vi "Exclude Path Options.vi"(8 "Error In":errorcluster, 11 "Path In":path) -> (0 "Error Out":errorcluster)   [LabVIEW 2010]
doc: "Use this template to build a standard state machine design pattern. Each state executes code and determines which state to transition to. Contrast this design pattern with the User Interface Event Handler pattern, in which code executes in response to user actions. Contrast this design pattern also with the Queued Message Handler pattern, in which each message handling code can queue zero or more new messages."
uses:
  Settings_option.ctl
panel:
  in  "System Key":string
  in  "EXCLUDE PATHS":path[](array[path])
  in  "Save":bool
  in  "Exit":bool
  # "OPTIONS"
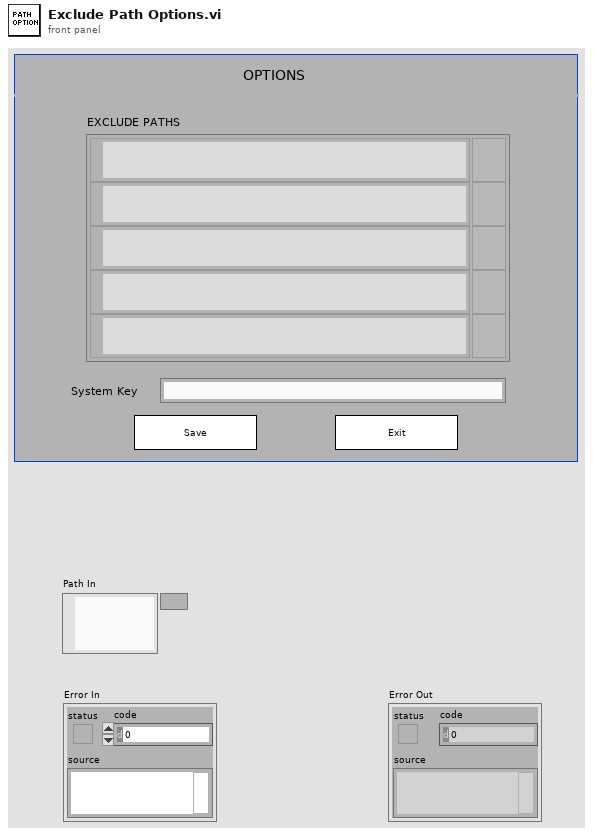
[diagram p1: front panel]
types:
  T1 = cluster{"Path In":path, "Exclude path":path[], "SystemKey":string}
  T2 = typedef "Settings_option.ctl" = enum16{"Poll", "Initialize", "Read", "Write", "Delete", "Exit"}
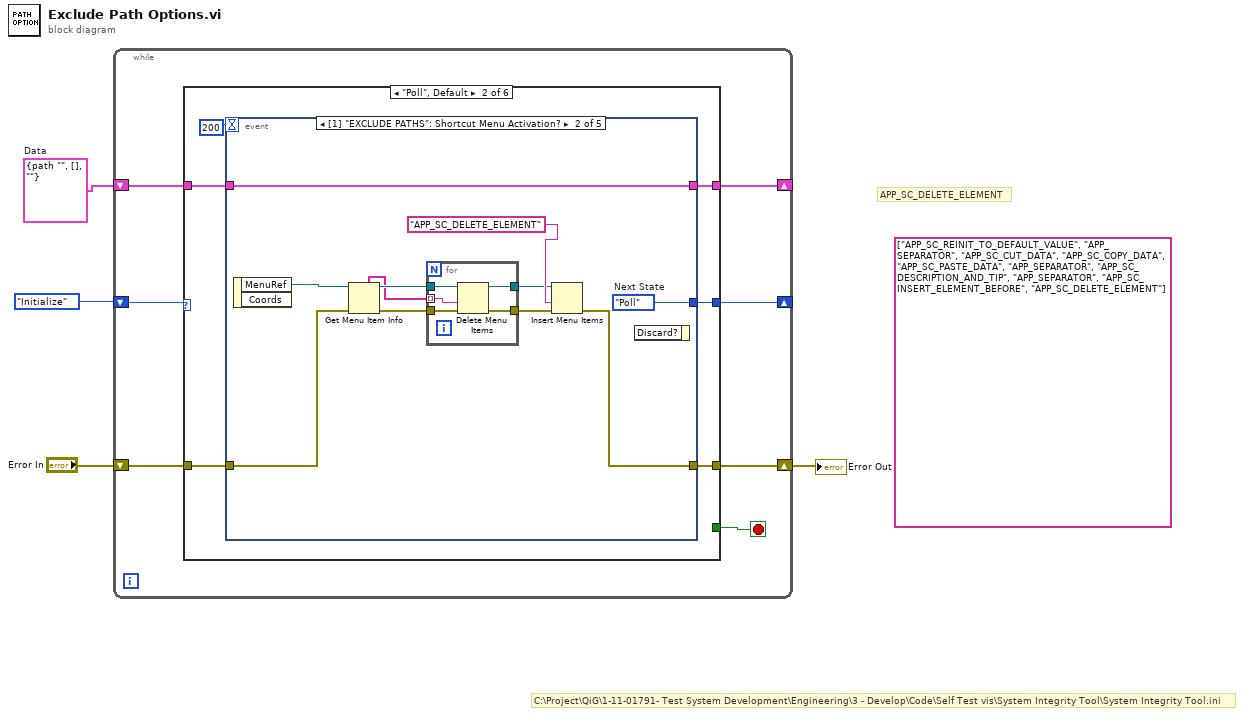
[diagram p0: block diagram]
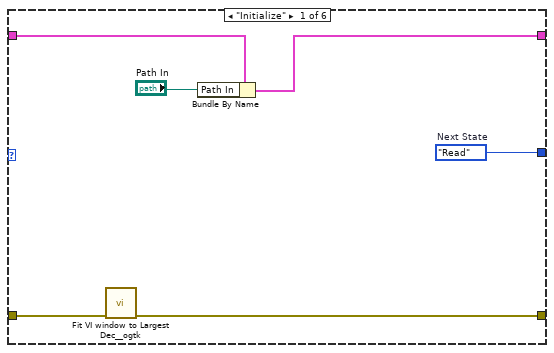
[diagram p2: hidden frame]
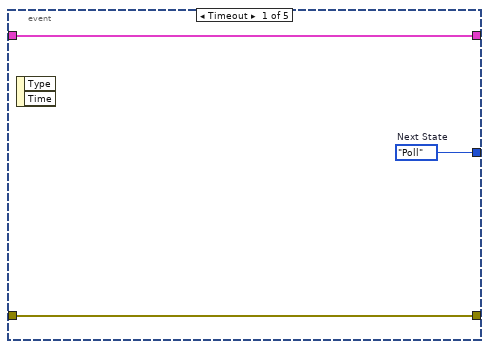
[diagram p3: hidden frame]
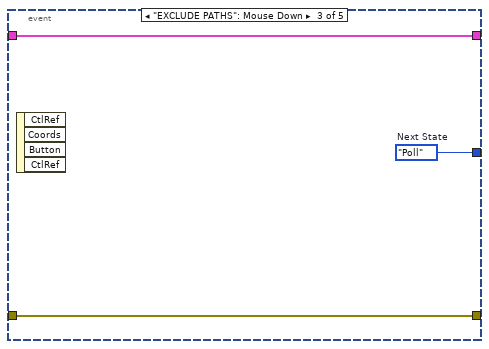
[diagram p4: hidden frame]
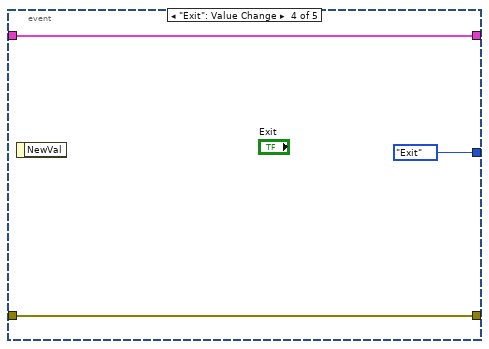
[diagram p5: hidden frame]
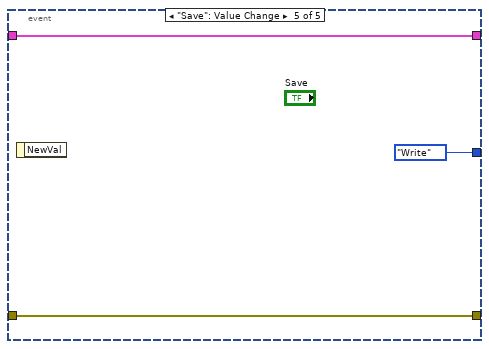
[diagram p6: hidden frame]
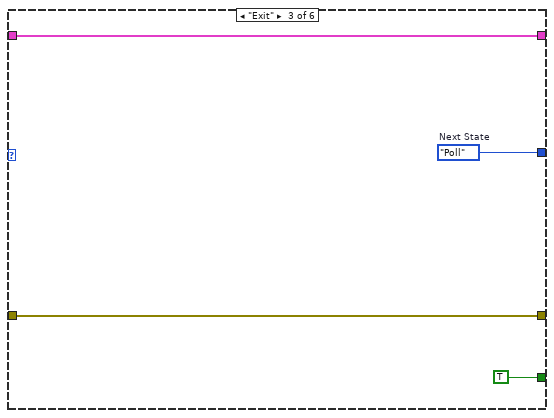
[diagram p7: hidden frame]
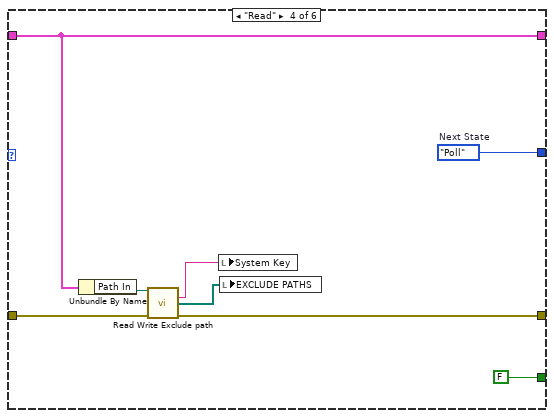
[diagram p8: hidden frame]
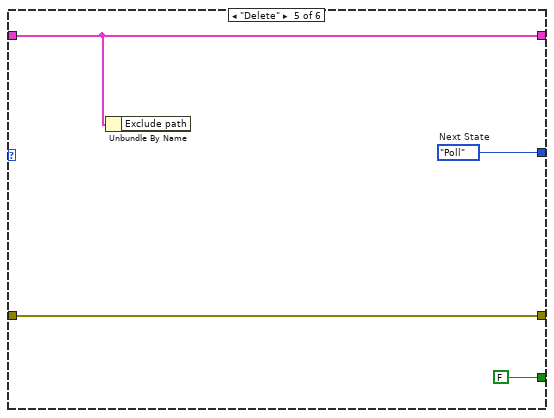
[diagram p9: hidden frame]
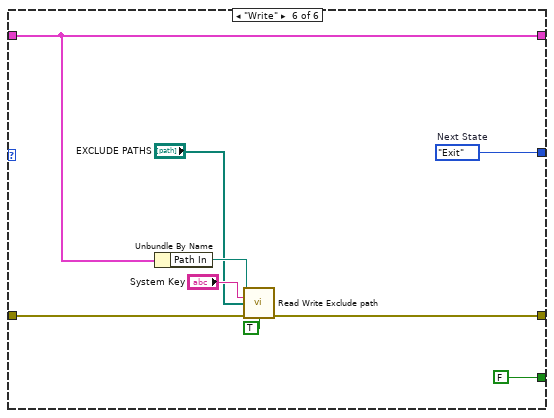
[diagram p10: hidden frame]
diagram:
  (unwired) string[] ["APP_SC_REINIT_TO_DEFAULT_VALUE", "APP_SEPARATOR", "APP_SC_CUT_DATA", "APP_SC_COPY_DATA", "APP_SC_PASTE_DATA", "APP_SEPARATOR", "APP_SC_DESCRIPTION_AND_TIP", "APP_SEPARATOR", "APP_SC_INSERT_ELEMENT_BEFORE", "APP_SC_DELETE_ELEMENT"] ("submenu tags 2")
  w1 = T1 {"Path In"=path "", "Exclude path"=[], "SystemKey"=""}  # Data
  # "APP_SC_DELETE_ELEMENT"
  # "C:\\Project\\QiG\\1-11-01791- Test System Development\\Engineering\\3 - Develop\\Code\\Self Test vis\\System Integrity Tool\\System Integrity Tool.ini"
  n1 = while {
    shift-right: [w10] -> _
    shift-left: Settings_option."Initialize" ("Beginning State") -> [w11]
    shift-right: [w7] -> w2
    shift-left: "Error In" -> [w8]
    shift-right: [w6] -> _
    shift-left: w1 -> [w5]
    stop <- w9 stop-if-true
    n2 = case shown="\"Poll\", Default" w11 {
      tunnel: [w17 w23 w55 w63 w67 w76] -> w10
      tunnel: [_ _ TRUE FALSE FALSE FALSE] -> w9
      tunnel: w8 -> [w16 w21 w53 w61 w64 w74]
      tunnel: [w15 w20 w53 w60 w64 w73] -> w7
      tunnel: [w13 w18 w52 w59 w65 w72] -> w6
      tunnel: w5 -> [w14 w19 w52 w59 w65 w72]
      frame "Initialize" {
        w17 = Settings_option."Read"  # Next State
        n3 = call "Fit VI window to Largest Dec__ogtk.vi"("error in (no error)"=w16) -> ("error out"=w15:errorcluster)  [unwired: 5 in, 1 out]
        n4 = Bundle By Name(cluster=w14, "Path In"="Path In") -> (w13:T1)
      }
      frame "Poll", Default {
        n5 = event shown="[1] \"EXCLUDE PATHS\": Shortcut Menu Activation?" {
          selector: _ -> [_ _ _ _ _]
          dyn-events: _ -> [_ _ _ _ _]
          timeout: 200 -> [_ _ _ _ _]
          tunnel: [w26 w37 w45 Settings_option."Exit" ("Next State") Settings_option."Write" ("Next State")] -> w23
          tunnel: [w25 w29 w44 w47 w50] -> w20
          tunnel: w21 -> [w25 w32 w44 w47 w50]
          tunnel: [w24 w36 w43 w46 w49] -> w18
          tunnel: w19 -> [w24 w36 w43 w46 w49]
          event Timeout {
            w26 = Settings_option."Poll"  # Next State
            n6 = event-data() -> ()  [unwired: 1 in, 2 out]
          }
          event "EXCLUDE PATHS": Shortcut Menu Activation? {
            w37 = Settings_option."Poll"  # Next State
            n7 = event-data() -> ("MenuRef"=w35:refnum<k9>)  [unwired: 1 in, 1 out]
            n8 = Get Menu Item Info(8:w32, 11:w35) -> (0:w33:errorcluster, 3:w34:refnum<k9>, 5:w31:string[])  [unwired: 1 in, 4 out]
            n9 = for {
              tunnel: w34 -> [w42]
              tunnel: w33 -> [w41]
              tunnel: w31 -> [w40] mode=indexing
              tunnel: [w39] -> w30
              tunnel: [w38] -> w27
              n10 = Delete Menu Items(6:w41, 7:w40, 9:w42) -> (0:w39:errorcluster, 3:w38:refnum<k9>)  [unwired: 1 in]
            }
            n11 = Insert Menu Items(6:w30, 7:"APP_SC_DELETE_ELEMENT", 9:w27) -> (0:w29:errorcluster)  [unwired: 3 in, 2 out]
            n12 = event-data() -> ()  [unwired: 2 in, 1 out]
          }
          event "EXCLUDE PATHS": Mouse Down {
            w45 = Settings_option."Poll"  # Next State
            n13 = event-data() -> ()  [unwired: 1 in, 4 out]
          }
          event "Exit": Value Change {
            n14 = event-data() -> ()  [unwired: 1 in, 1 out]
          }
          event "Save": Value Change {
            n15 = event-data() -> ()  [unwired: 1 in, 1 out]
          }
        }
      }
      frame "Exit" {
        w55 = Settings_option."Poll"  # Next State
      }
      frame "Read" {
        w63 = Settings_option."Poll"  # Next State
        n16 = Unbundle By Name(w59) -> ("Path In"=w58:path)
        n17 = call "Read Write Exclude path.vi"("path In"=w58, "Error In"=w61) -> ("Key out"=w57:string, "Exclude Path Out"=w56:path[], "Error Out"=w60:errorcluster)  [unwired: 10 in, 1 out]
        n18 = local write "System Key"(w57) -> ()
        n19 = local write "EXCLUDE PATHS"(w56) -> ()
      }
      frame "Delete" {
        w67 = Settings_option."Poll"  # Next State
        n20 = Unbundle By Name(w65) -> ()  [unwired: 1 out]
      }
      frame "Write" {
        w76 = Settings_option."Exit"  # Next State
        n21 = Unbundle By Name(w72) -> ("Path In"=w71:path)
        n22 = call "Read Write Exclude path.vi"("path In"=w71, "Key In"="System Key", "Exclude Path In"="EXCLUDE PATHS", "Error In"=w74, "Write?"=TRUE) -> ("Error Out"=w73:errorcluster)  [unwired: 7 in, 3 out]
      }
    }
  }
  "Error Out" <- w2
